vi "Check If Trace Exists.vi"(8 "error in (no error)":errorcluster, 10 "Trace Name":refnum<k21>, 11 "Database":path=path "\\\\localhost\\c__data") -> (0 "error out":errorcluster, 2 "Exist?":bool, 3 "dup Database":path=path "\\\\localhost\\c__data")   [LabVIEW 2024]
doc: "Checks if a trace exists in the database."
uses:
  <vilib>/lvdsc/NI_DSC.lvlib
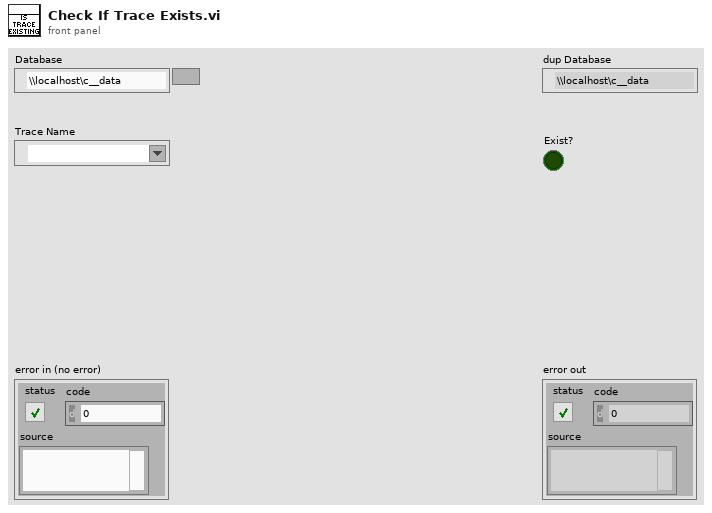
[diagram p1: front panel]
types:
  T1 = enum16{"Analog", "Discrete", "BitArray", "String", "Undefined", "Variant"}
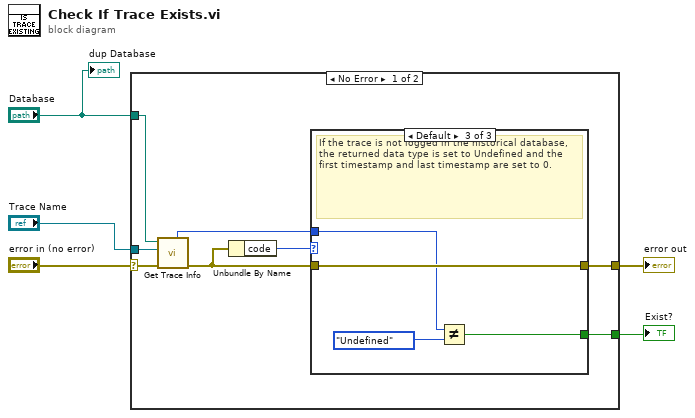
[diagram p0: block diagram]
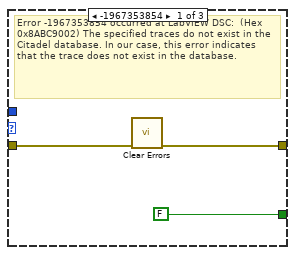
[diagram p2: hidden frame]
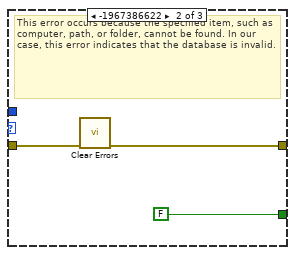
[diagram p3: hidden frame]
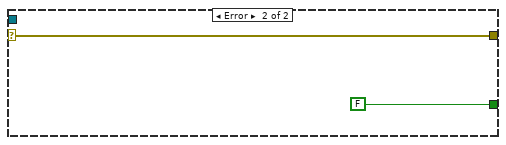
[diagram p4: hidden frame]
diagram:
  n1 = case shown="No Error" "error in (no error)" {
    selector: "error in (no error)" -> [w13 w25]
    tunnel: [w10 w25] -> w5
    tunnel: [w9 FALSE ("Exist?")] -> w3
    tunnel: "Database" -> [w7 _]
    tunnel: "Trace Name" -> [w6 _]
    frame No Error {
      n2 = call <vilib>:"Get Trace Info.vi"("error in (no error)"=w13, "trace name"=w6, "database URL"=w7) -> ("error out"=w11:errorcluster, "data type"=w8:T1)  [unwired: 4 in, 3 out]
      n3 = Unbundle By Name(w11) -> ("code"=w12:i32)
      n4 = case shown="Default" w12 {
        tunnel: w11 -> [w15 w18 w23]
        tunnel: [w14 w17 w23] -> w10
        tunnel: [FALSE ("Exist?") FALSE ("Exist?") w20] -> w9
        tunnel: w8 -> [_ _ w22]
        frame -1967353854 {
          # "Error -1967353854 occurred at LabVIEW DSC:  (Hex 0x8ABC9002) The specified traces do not exist in the Citadel database. In our case, this error indicates that the trace does not exist in the database."
          n5 = call <vilib>:"Clear Errors.vi"("error in (no error)"=w15) -> ("error out"=w14:errorcluster)  [unwired: 5 in, 1 out]
        }
        frame -1967386622 {
          # "This error occurs because the specified item, such as computer, path, or folder, cannot be found. In our case, this error indicates that the database is invalid."
          n6 = call <vilib>:"Clear Errors.vi"("error in (no error)"=w18) -> ("error out"=w17:errorcluster)  [unwired: 5 in, 1 out]
        }
        frame Default {
          # "If the trace is not logged in the historical database, the returned data type is set to Undefined and the first timestamp and last timestamp are set to 0."
          n7 = Not Equal?(x=w22, y=T1."Undefined") -> (x != y?=w20:bool)
        }
      }
    }
    frame Error {
    }
  }
  "error out" <- w5
  "Exist?" <- w3
  "dup Database" <- "Database"
